vi "TestClone.vi"() -> ()   [LabVIEW 2014, in "EventModule.lvlib"]
uses:
  EventModule.lvlib
  EventPlugins/EventPluginBaseClass/TypeDefs/clEvtConfig.ctl
  PublicAPI/Arguments/Requests/dblEvtParams.ctl
  PublicAPI/Arguments/Requests/dblTimeArray.ctl
  EventPlugins/EventPluginBaseClass/TypeDefs/clEvtReportArray.ctl
  EventPlugins/EventPluginBaseClass/TypeDefs/clEvtReport.ctl
  EventPlugins/EventPluginBaseClass/TypeDefs/dblEvtSignalArray.ctl
  TestInfo.ctl
  <userlib>/NIST/ModuleAdminLib/ModuleAdmin/ModuleAdmin.lvclass
  PublicAPI/Arguments/Broadcasts/clDidInit.ctl
  <userlib>/NIST/ModuleAdminLib/ModuleAdmin/ModuleAdmin.lvclass/ModuleAdmin.ctl
  PublicAPI/Arguments/Requests/clStopArgument.ctl
  PublicAPI/Arguments/Broadcasts/clStatUpdate.ctl
  PublicAPI/Arguments/Broadcasts/clErrorRpt.ctl
  <userlib>/NIST/ModuleAdminLib/ModuleAdmin/Accessors/Read CloneRegRef.vi
  <vilib>/Analysis/1siggen.llb/Ramp Pattern by Delta.vi
  <userlib>/NIST/ModuleAdminLib/CloneRegistration/CloneRegistration.lvclass
  EventPlugins/EventPluginBaseClass/EventPluginBaseClass.lvclass
  <vilib>/Analysis/NI_AALBase.lvlib
panel:
  in  "Show Panel":bool=TRUE
  in  "End Time":dbl
  in  "Start Time":dbl
  in  "Plugin Type":u16(ring) items=["C37.118.1", "Frequency Ramp", "Modulation", "Ringdown", "Steady State", "Step", "60255Harm", "User1", "User2"]
  in  "btnGetEvtSignal":bool
  out "dblEventSignalArray":T1
  out "PathToPluginIniFileReport":path=path "P:/Framework/Events/EventPlugins/SSEvtPlugin/SteadyStateEventPlugin.ini"
  in  "btnReadPathToPlugin":bool
  in  "btnGetEvtReportArray":bool
  out "clEvtReportArray":T2 {"Synx" format="%#_4g"}
  in  "btnReadEvtParams":bool
  in  "btnWriteEvtParams":bool
  in  "btnReadTimeArray":bool
  in  "btnWriteTimeArray":bool
  out "dblTimeArrayReport":T4
  out "dblEvtParamsReport":T5
  out "dblTimeArray":T4=[0.0, 0.05, 0.1, 0.15000000000000002, 0.2]
  in  "dblEvtParams":T5=[[0.0, 0.34657, 0.69677, 1.297, 1.4569, 6.0606, 7.2288, 8.9506, 11.705, 18.574], [1000.0, 24.879, 55.751, 46.204, 36.867, 1.995, 0.82578, 1.5487, 1.8652, 1.6268], [0.0, 1.876, 0.28983, 1.5993, 2.6728, 3.9286, 1.2558, 3.3379, 3.6506, 7.1708], [0.0, -67.696, -60.912, 99.138, -123.76, 176.38, -149.46, -106.27, -18.535, -59.29], [0.0, 0.0, 0.58767, 0.6985, 1.3263, 2.7275, 7.1783, 8.122, 14.704, 15.622], [200.0, 31.231, 41.605, 48.38, 1.6511, 0.84175, 2.671, 0.64619, 0.78365, 0.6061], [0.0, 6.2405, 2.3071, 0.28998, 1.025, 3.6069, 15.284, 3.3041, 2.4034, 2.5242], [0.0, 180.0, 37.683, 113.63, 41.526, 4.7072, 5.0124, -177.41, -50.759, 41.697], [568.0, 0.0, 0.0, 0.0, 0.0, 0.0, 0.0, 0.0, 0.0, 0.0], [0.0, 0.0, 0.0, 0.0, 0.0, 0.0, 0.0, 0.0, 0.0, 0.0], [0.0, 0.0, 0.0, 0.0, 0.0, 0.0, 0.0, 0.0, 0.0, 0.0], [0.0, 0.0, 0.0, 0.0, 0.0, 0.0, 0.0, 0.0, 0.0, 0.0], [0.0, 0.0, 0.0, 0.0, 0.0, 0.0, 0.0, 0.0, 0.0, 0.0]]
  out "clEvtConfigReport":T6={"T0(UTC)"=0.0, "F0"=0.0, "Fs"=60, "FSamp"=0, "bPosSeq"=FALSE}
  in  "btnReadEvtConfig":bool
  in  "clEvtConfig":T6={"T0(UTC)"=0.0, "F0"=60.0, "Fs"=60, "FSamp"=960, "bPosSeq"=FALSE}
  in  "btnWriteEvtConfig":bool
  in  "btnLoadPlugin":bool
  in  "btnRemove":bool
  out "Status Log":string
  out "Active Modules (Array)":string[](array[string])
  in  "btnAdd":bool
  in  "btnStop":bool
  in  "Select Module":i32(ring)=-1 caption="Select Module to send Request" items=["All"=-1]
  # "Hidden"
  # "Visible"
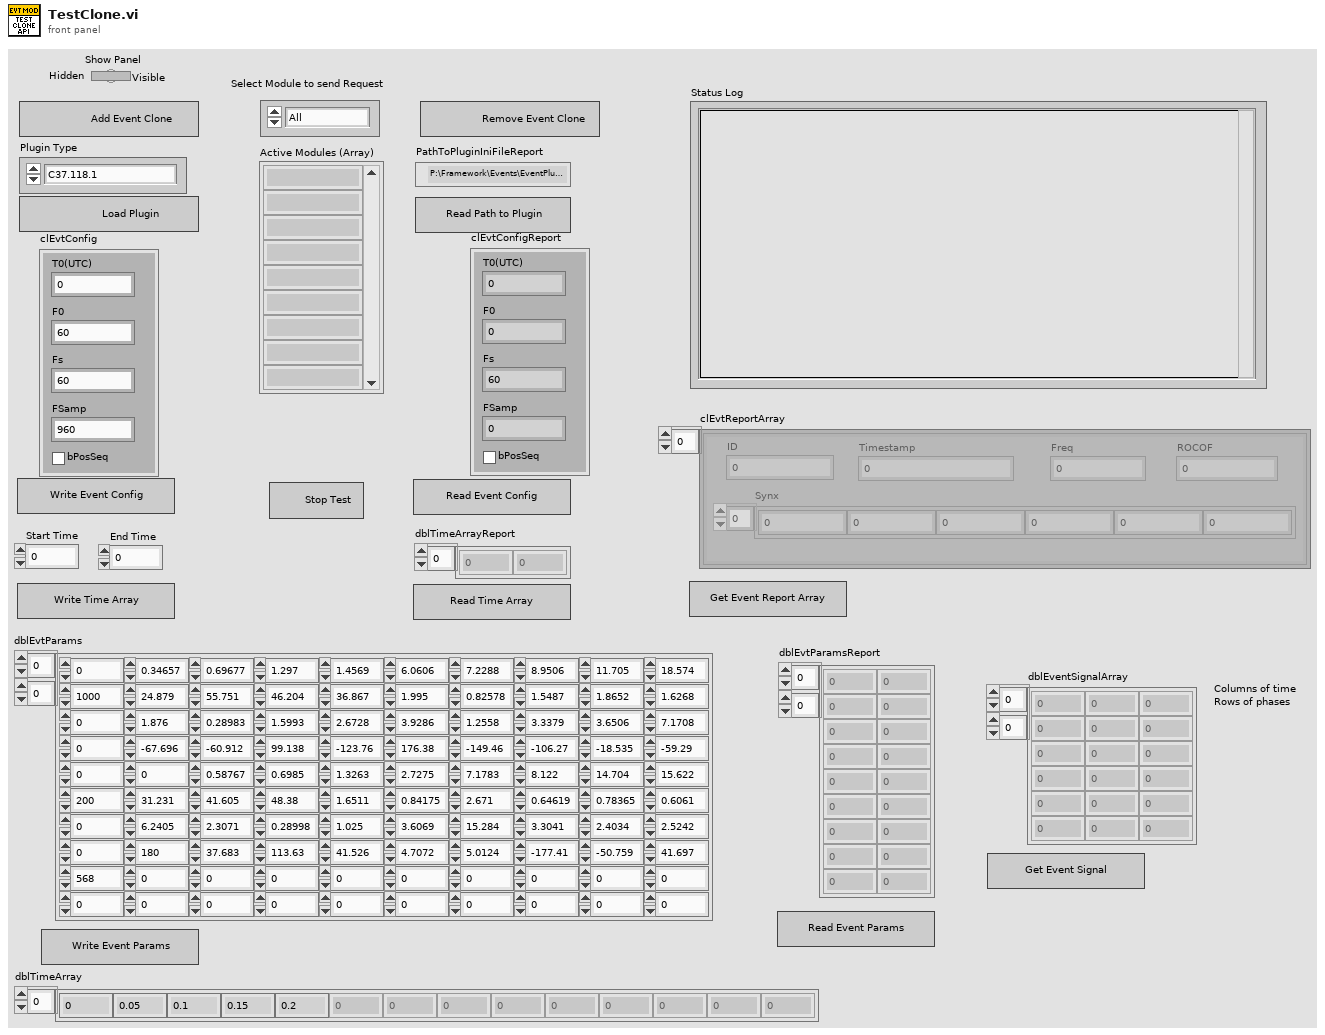
[diagram p1: front panel]
types:
  T1 = typedef "EventPlugins.lvlib/EventPluginBaseClass.lvclass/dblEvtSignalArray.ctl" = dbl[][]
  T2 = typedef "EventPlugins.lvlib/EventPluginBaseClass.lvclass/clEvtReportArray.ctl" = T3[]
  T3 = typedef "EventPlugins.lvlib/EventPluginBaseClass.lvclass/clEvtReport.ctl" = cluster{"Timestamp":dbl, "Synx":cdb[], "Freq":dbl, "ROCOF":dbl, "ID":i16}
  T4 = typedef "EventModule.lvlib/dblTimeArray.ctl" = dbl[]
  T5 = typedef "EventModule.lvlib/dblEvtParams.ctl" = dbl[][]
  T6 = typedef "EventPlugins.lvlib/EventPluginBaseClass.lvclass/clEvtConfig.ctl" = cluster{"T0(UTC)":dbl, "F0":dbl, "Fs":i32, "FSamp":u32, "bPosSeq":bool}
  T7 = typedef "EventModule.lvlib/TestInfo.ctl" = cluster{"PluginIniFilePaths":path[]}
  T8 = typedef "EventModule.lvlib/clBroadcastEvents.ctl" = cluster{"DidInit":refnum<user-event>, "StatusUpdate":refnum<user-event>, "ErrorReport":refnum<user-event>, "DidStop":refnum<user-event>, "ReadEvtConfig":refnum<user-event>, "ReadTimeArray":refnum<user-event>, "ReadEvtParams":refnum<user-event>, "GetEvtReportArray":refnum<user-event>, "ReadPathToPlugin":refnum<user-event>, "GetEvtSignal":refnum<user-event>, "ReadBusNumber":refnum<user-event>}
  T9 = typedef "EventModule.lvlib/clDidInit.ctl" = cluster{"Init?":bool, "ModuleAdmin":refnum<class "ModuleAdmin.lvclass">}
  T10 = typedef "EventModule.lvlib/clStopArgument.ctl" = cluster{"Exit via Stop Module Req?":bool, "Wait for Module to stop?":bool, "ModuleAdmin":refnum<class "ModuleAdmin.lvclass">}
  T11 = typedef "EventModule.lvlib/clStatUpdate.ctl" = cluster{"Status":string}
  T12 = typedef "EventModule.lvlib/clErrorRpt.ctl" = cluster{"error":errorcluster, "AdditionalInfo":string}
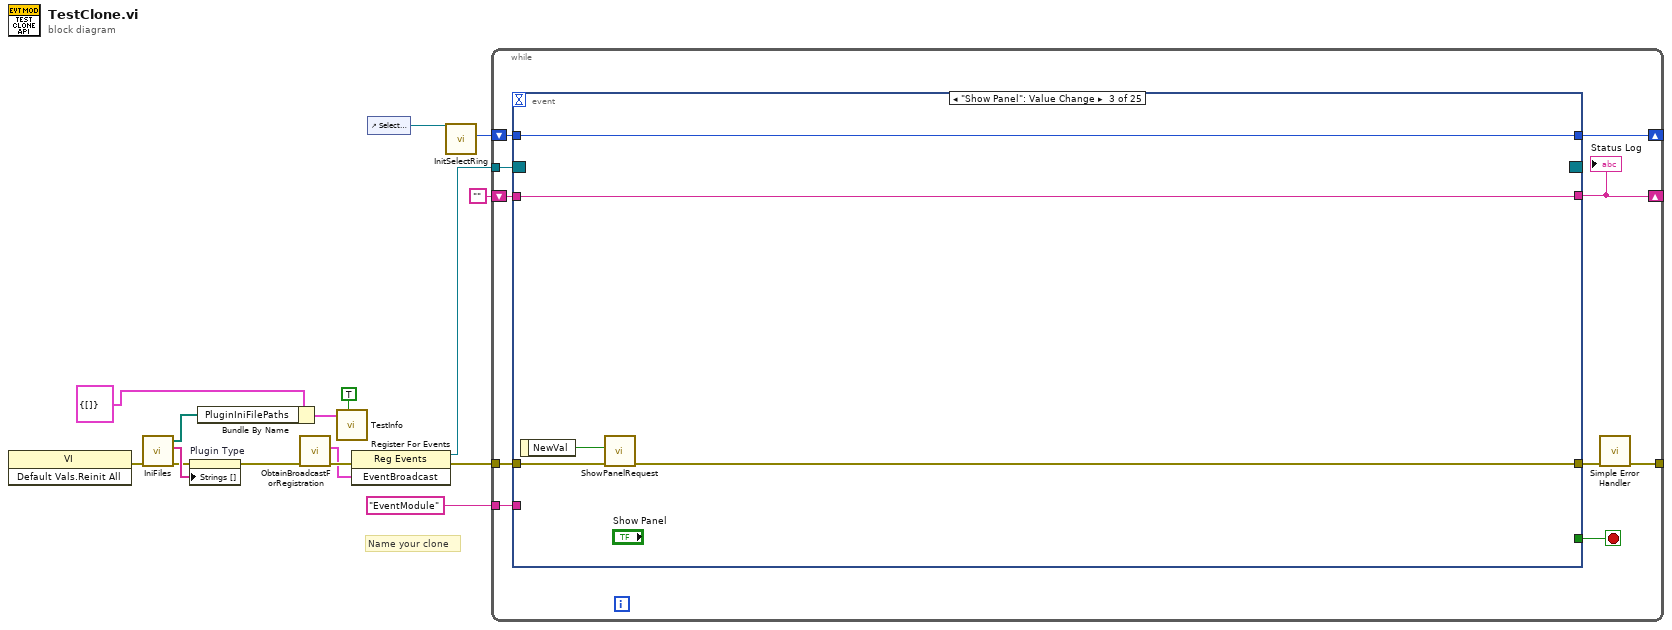
[diagram p0: block diagram]
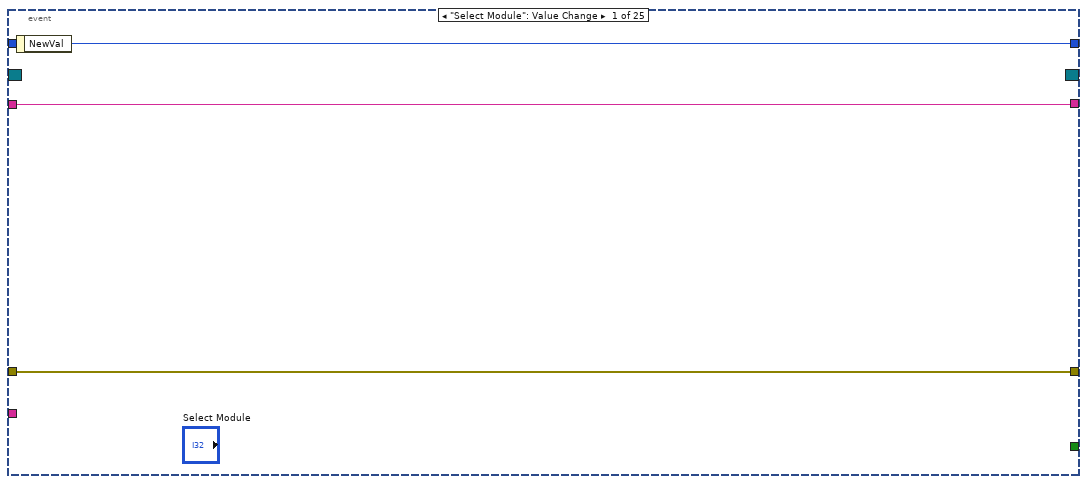
[diagram p2: hidden frame]
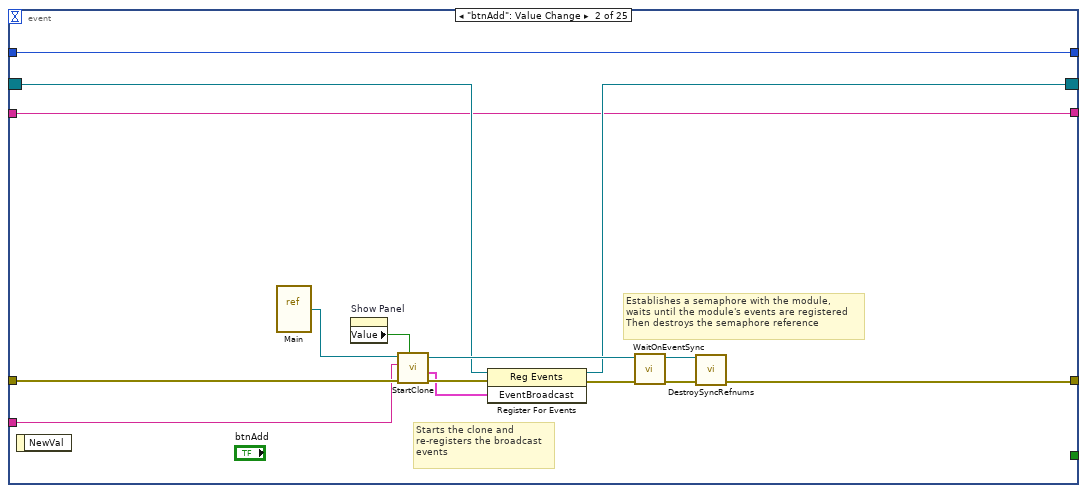
[diagram p3: hidden frame]
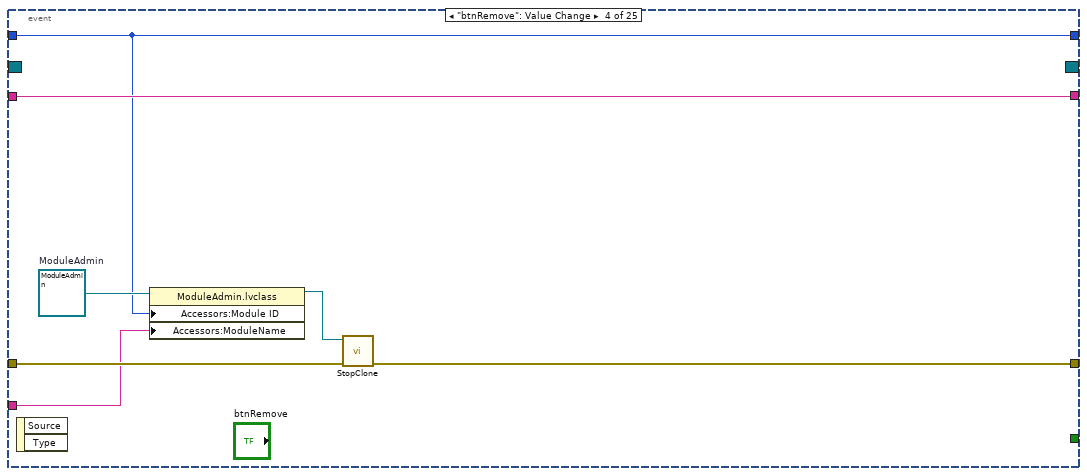
[diagram p4: hidden frame]
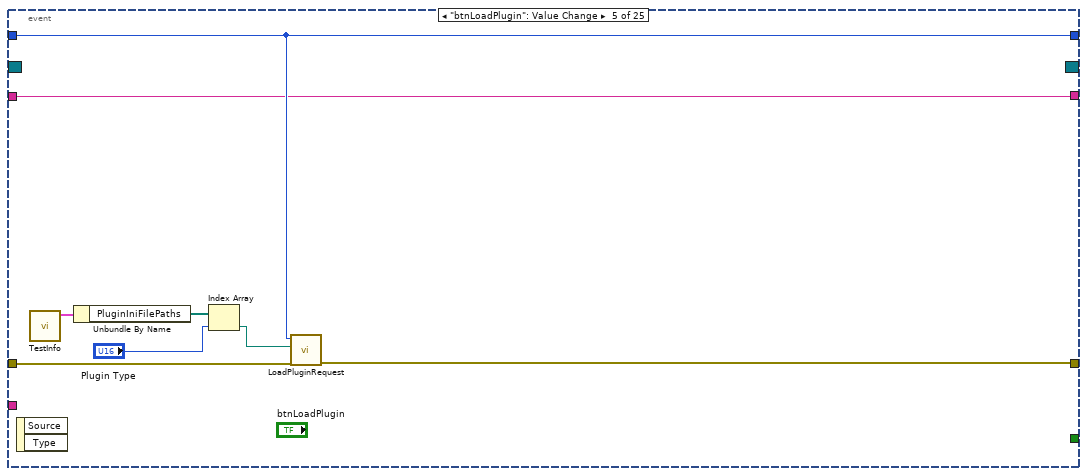
[diagram p5: hidden frame]
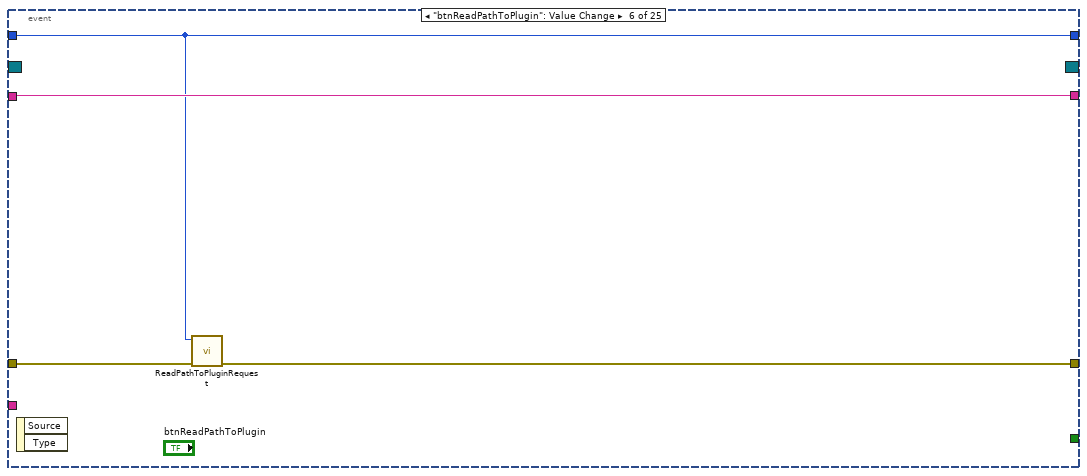
[diagram p6: hidden frame]
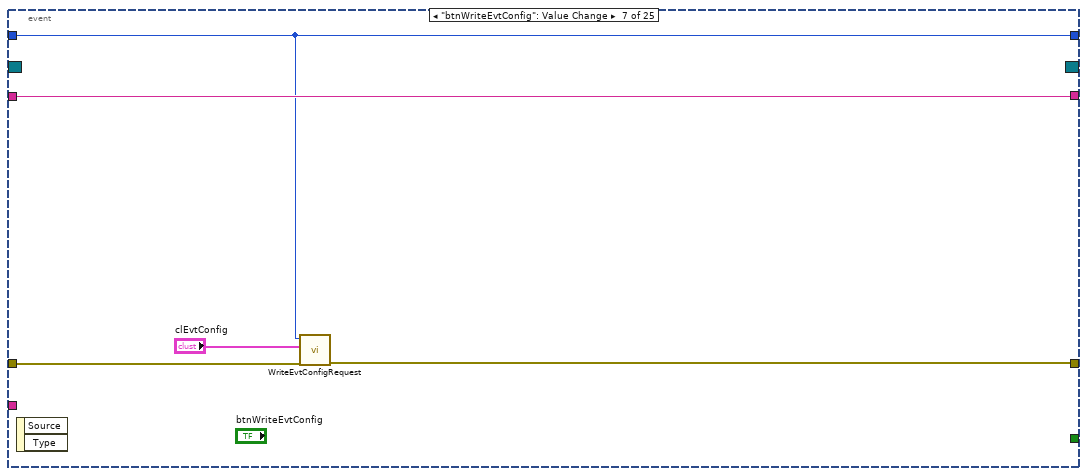
[diagram p7: hidden frame]
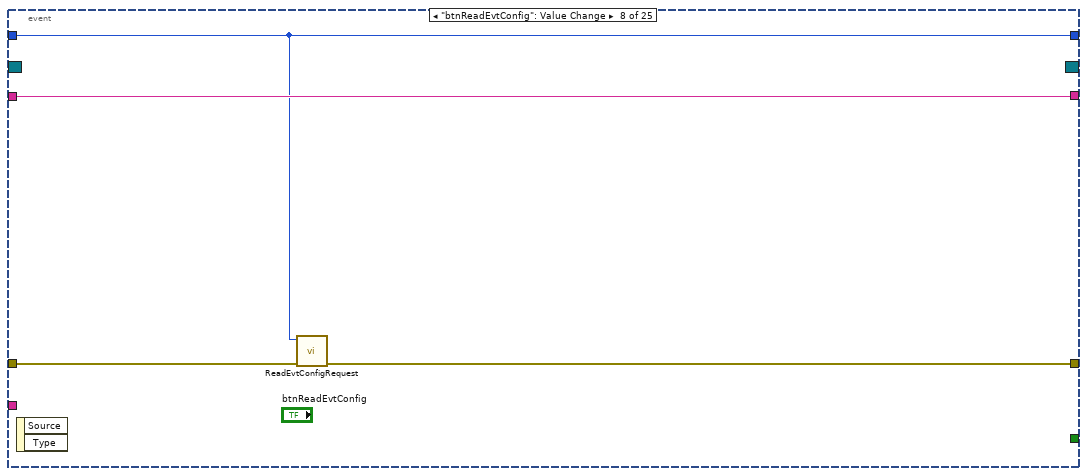
[diagram p8: hidden frame]
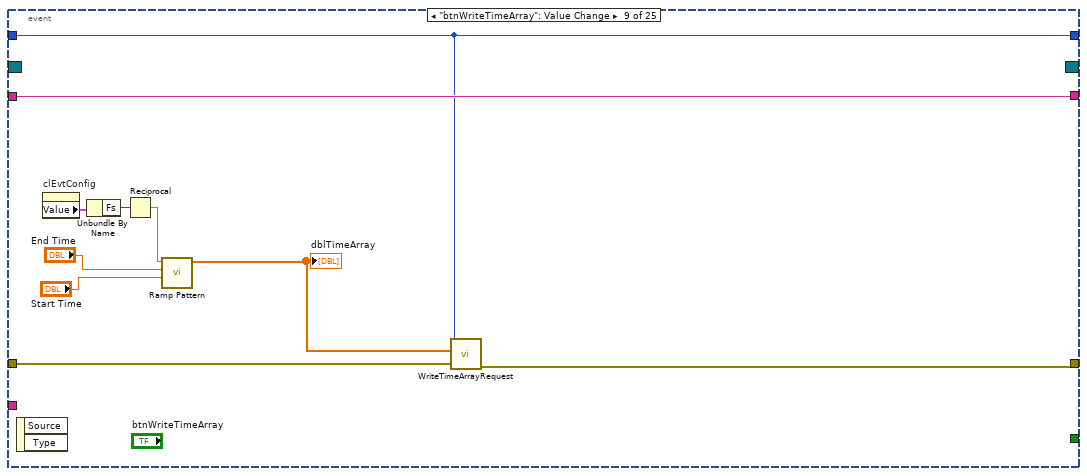
[diagram p9: hidden frame]
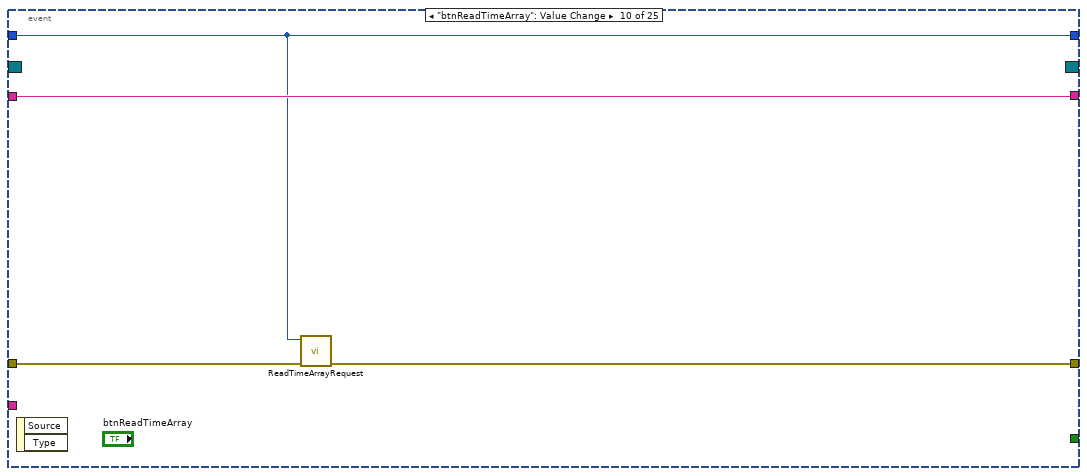
[diagram p10: hidden frame]
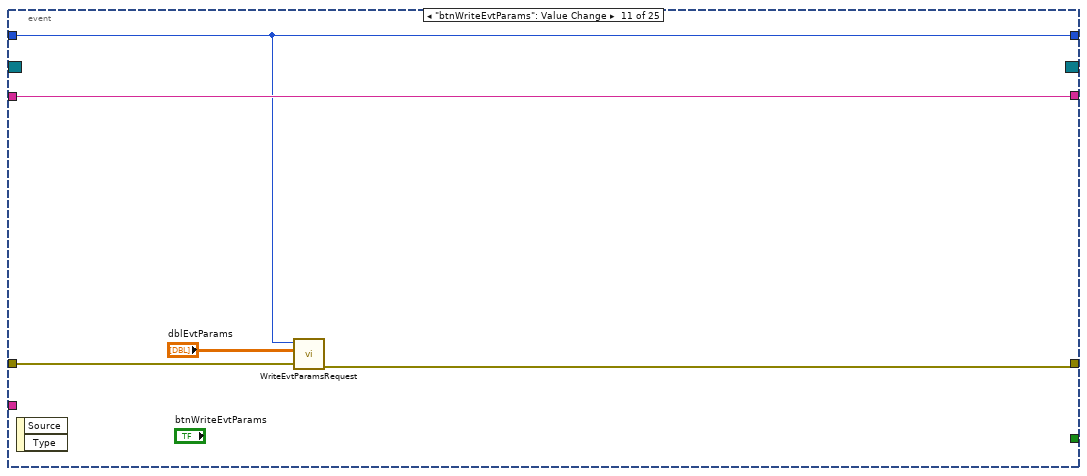
[diagram p11: hidden frame]
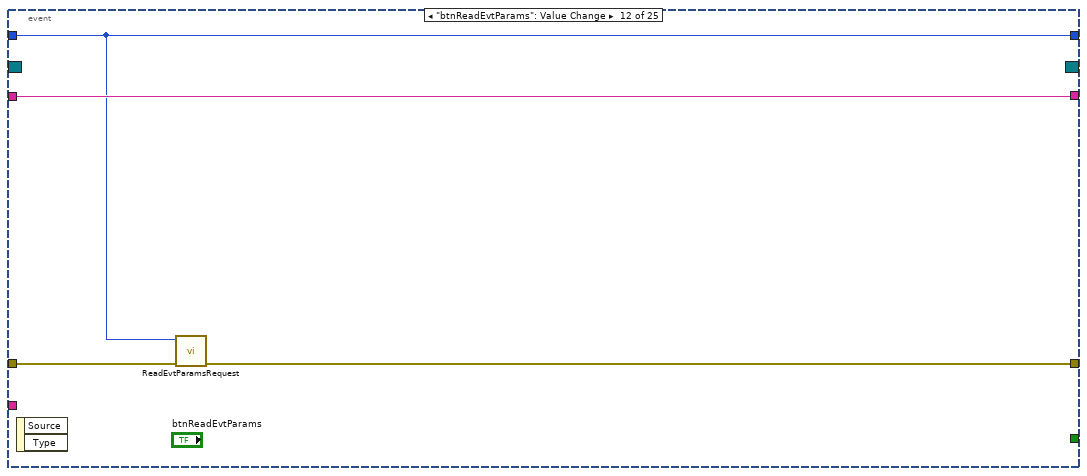
[diagram p12: hidden frame]
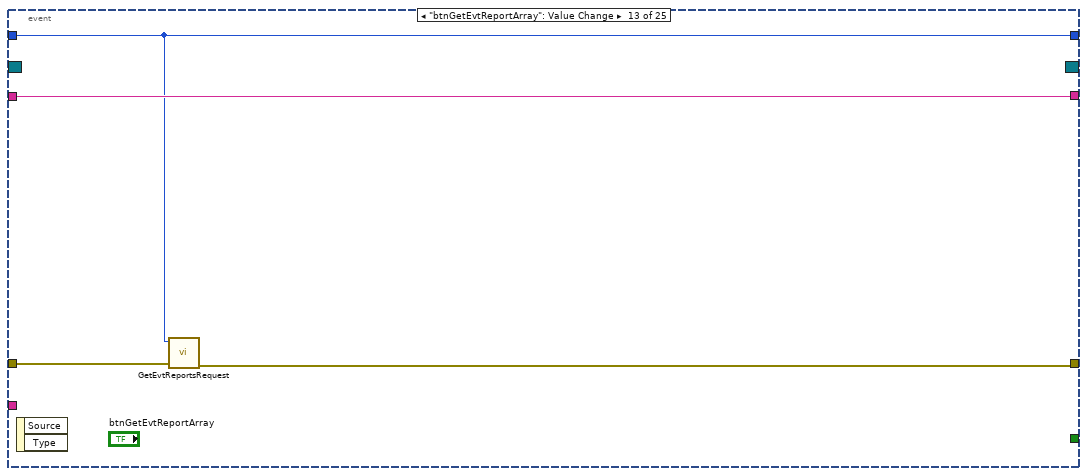
[diagram p13: hidden frame]
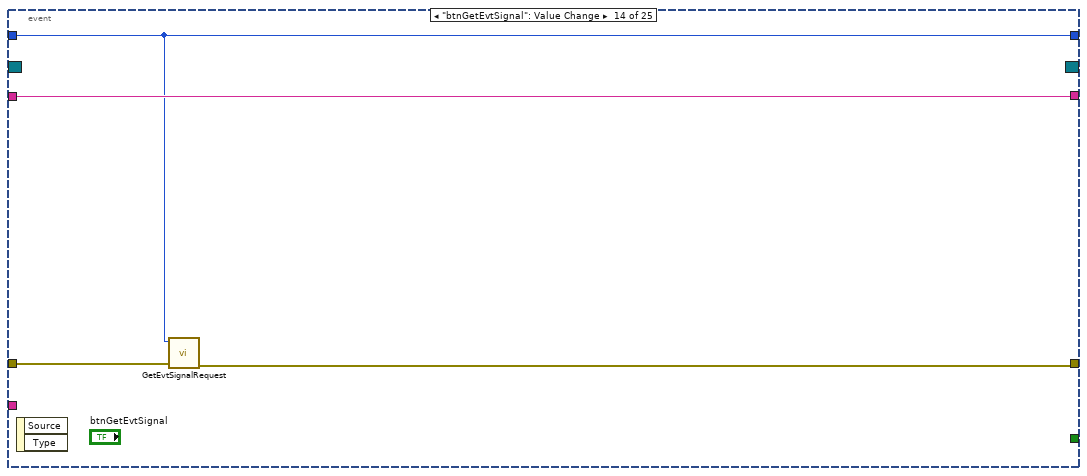
[diagram p14: hidden frame]
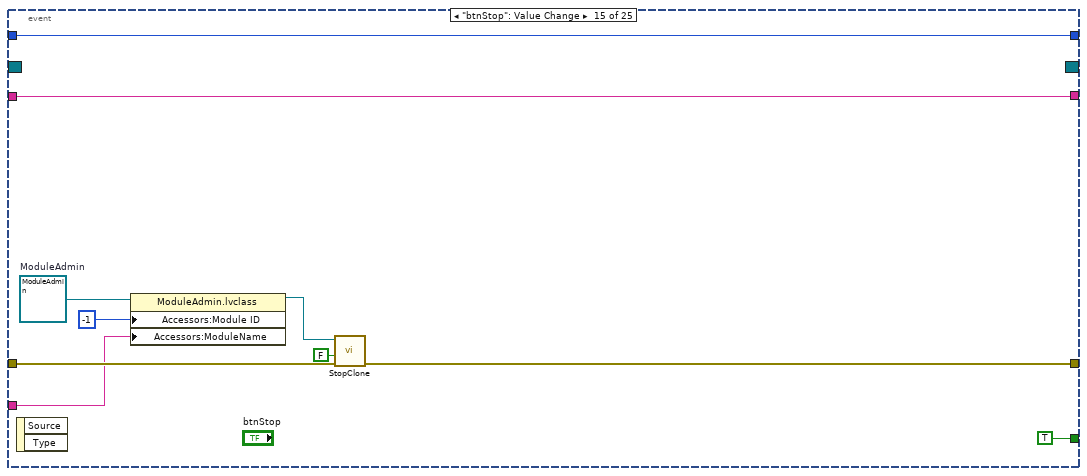
[diagram p15: hidden frame]
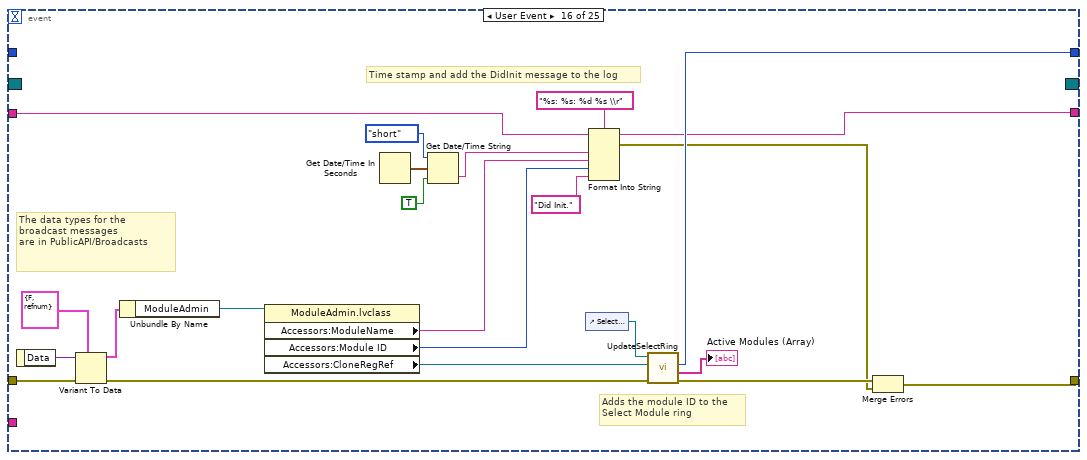
[diagram p16: hidden frame]
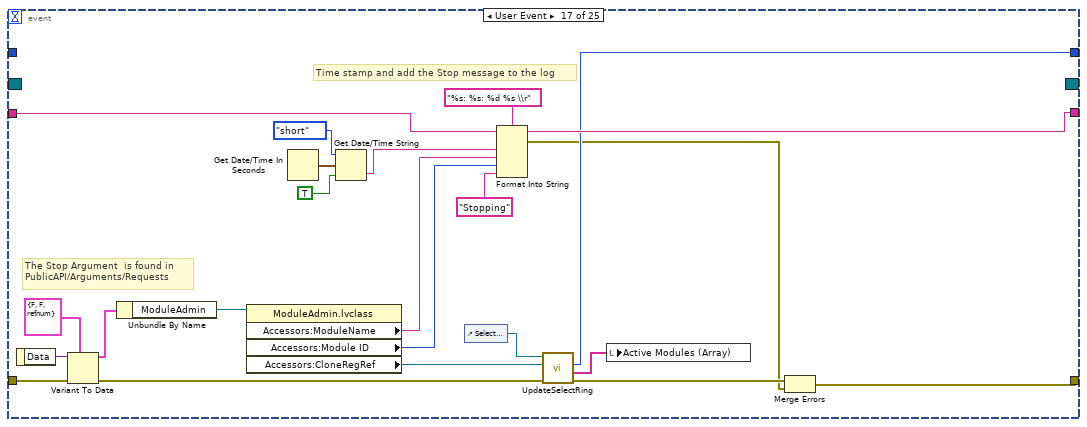
[diagram p17: hidden frame]
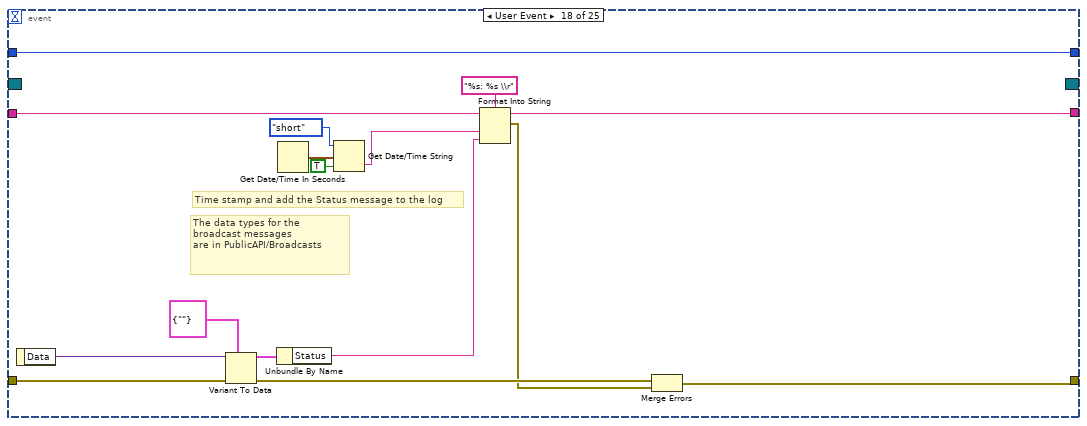
[diagram p18: hidden frame]
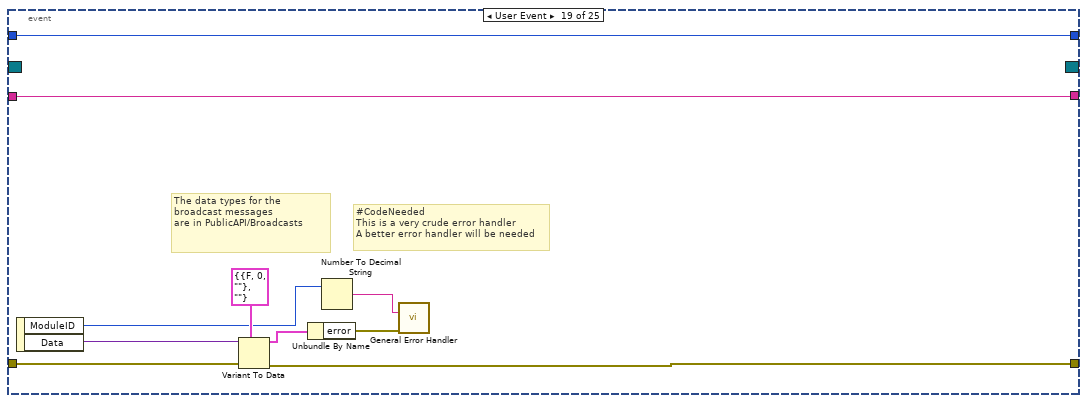
[diagram p19: hidden frame]
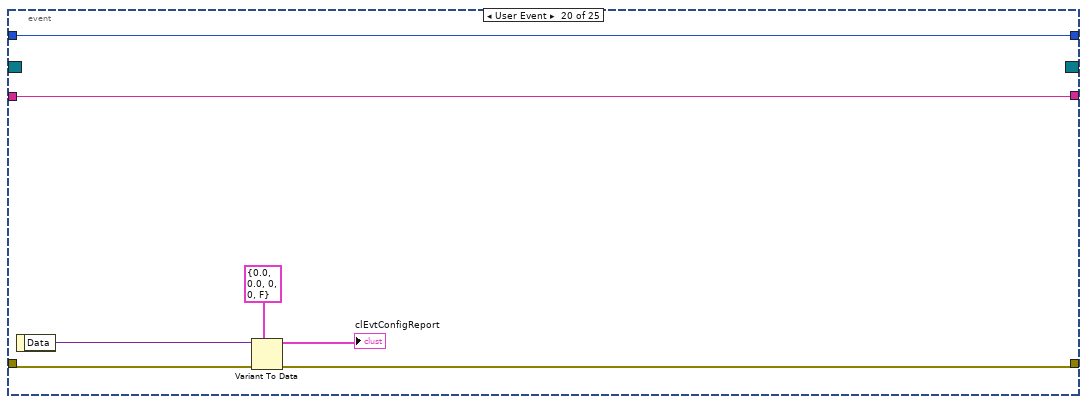
[diagram p20: hidden frame]
diagram:
  # "Name your clone"
  n1 = invoke class="VI" method="Default Vals.Reinit All"() -> (error out=w8:errorcluster)  [unwired: 3 in, 2 out]
  n2 = call "IniFiles.vi"("error in"=w8) -> ("error out"=w6:errorcluster, "Types"=w7:string[], "IniFilePaths"=w3:path[])  [unwired: 8 in]
  n3 = property on="Plugin Type" class="Ring (strict)"(error in=w6, "Strings []"=w7) -> (error out=w5:errorcluster)  [unwired: 1 in, 1 out]
  n4 = Bundle By Name(cluster=T7 {"PluginIniFilePaths"=[]} ("TestInfo"), "PluginIniFilePaths"=w3) -> (w2:T7)
  n5 = call "ObtainBroadcastForRegistration.vi"("error in (no error)"=w5) -> ("error out"=w14:errorcluster, "EventBroadcast"=w13:T8)  [unwired: 9 in]
  n6 = call "TestInfo.vi"("Set (f)"=TRUE, "TestInfo"=w2) -> ()  [unwired: 9 in, 1 out]
  n7 = register-events(error in=w14, w13) -> (reference out=w11:refnum<event-registration>, error out=w12:errorcluster)  [unwired: 1 in]
  n8 = control-ref of="Select Module"() -> (w16:refnum<vi>)
  n9 = call "InitSelectRing.vi"("Ring Refnum"=w16) -> ("Module Ring Value"=w15:i32)  [unwired: 9 in, 1 out]
  n10 = while {
    shift-right: [w25] -> _
    shift-left: w15 -> [w26]
    tunnel: w12 -> [w23]
    tunnel: w11 -> [w20]
    tunnel: [w21] -> _
    shift-right: [w19] -> _
    shift-left: "" -> [w18]
    tunnel: "EventModule" ("ModuleName") -> [w17]
    stop <- w24 stop-if-true
    n11 = event shown="[2] \"Show Panel\": Value Change" {
      selector: w20 -> [_ w35 _ _ _ _ _ _ _ _ _ _ _ _ _ _ _ _ _ _ _ _ _ _ _]
      dyn-events: [_ w34 _ _ _ _ _ _ _ _ _ _ _ _ _ _ _ _ _ _ _ _ _ _ _] -> _
      timeout: _ -> [_ _ _ _ _ _ _ _ _ _ _ _ _ _ _ _ _ _ _ _ _ _ _ _ _]
      tunnel: w26 -> [_ w44 w45 w51 w63 w65 w70 w74 w84 w90 w93 w98 w101 w105 w118 _ _ w180 w182 w191 w199 w206 w213 w220 w228]
      tunnel: [w29 w44 w45 w51 w63 w65 w70 w74 w84 w90 w93 w98 w101 w105 w118 w136 w151 w180 w182 w191 w199 w206 w213 w220 w228] -> w25
      tunnel: [_ _ _ _ _ _ _ _ _ _ _ _ _ _ TRUE _ _ _ _ _ _ _ _ _ _] -> w24
      tunnel: w23 -> [w27 w43 w49 w55 w64 w67 w72 w76 w87 w89 w96 w99 w104 w108 w116 w141 w160 w177 w189 w194 w204 w208 w217 w225 w232]
      tunnel: [w27 w36 w47 w54 w62 w66 w69 w75 w86 w88 w94 w97 w103 w107 w114 w124 w148 w168 w188 w193 w203 w209 w215 w224 w231] -> w22
      tunnel: [w28 w32 w46 w56 w61 w68 w73 w77 w85 w91 w95 w100 w102 w106 w113 w128 w157 w171 w181 w192 w198 w207 w214 w221 w229] -> w19
      tunnel: w18 -> [w28 w32 w46 w56 w61 w68 w73 w77 w85 w91 w95 w100 w102 w106 w113 w127 w158 w179 w181 w192 w198 w207 w214 w221 w229]
      tunnel: w17 -> [_ w31 _ w52 _ _ _ _ _ _ _ _ _ _ w110 _ _ _ _ _ _ _ _ _ _]
      event "Select Module": Value Change {
        n12 = event-data() -> ("NewVal"=w29:i32)  [unwired: 1 in]
      }
      event "btnAdd": Value Change {
        # "Establishes a semaphore with the module,\nwaits until the module's events are registered\nThen destroys the semaphore reference"
        # "Starts the clone and\nre-registers the broadcast \nevents"
        n13 = event-data() -> ()  [unwired: 1 in, 1 out]
        n14 = vi-ref "Main.vi"() -> (w33:refnum<vi>)
        n15 = property on="Show Panel" class="Bool (strict)"() -> ("Value"=w30:bool)  [unwired: 2 in, 2 out]
        n16 = call "StartClone.vi"("ShowPanel? (f)"=w30, "error in (no error)"=w43, "ModuleName"=w31, "VI Refnum"=w33) -> ("error out"=w42:errorcluster, "clBroadcastEvents"=w37:T8, "ModuleAdmin"=w39:refnum<class "ModuleAdmin.lvclass">)  [unwired: 5 in]
        n17 = register-events(reference=w35, error in=w42, w37) -> (reference out=w34:refnum<event-registration>, error out=w41:errorcluster)
        n18 = call <userlib>:"WaitOnEventSync.vi"("error in (no error)"=w41, "ModuleAdmin"=w39) -> ("error out"=w40:errorcluster, "ModuleAdmin"=w38:refnum<class "ModuleAdmin.lvclass">)  [unwired: 8 in]
        n19 = call <userlib>:"DestroySyncRefnums.vi"("error in (no error)"=w40, "ModuleAdmin"=w38) -> ("error out"=w36:errorcluster)  [unwired: 9 in]
      }
      event "Show Panel": Value Change {
        n20 = event-data() -> ("NewVal"=w48:bool)  [unwired: 1 in]
        n21 = call "ShowPanelRequest.vi"("error in (no error)"=w49, "ShowPanel?"=w48) -> ("error out"=w47:errorcluster)  [unwired: 9 in]
      }
      event "btnRemove": Value Change {
        w53 = refnum<class "ModuleAdmin.lvclass"> refnum  # ModuleAdmin
        n22 = event-data() -> ()  [unwired: 1 in, 2 out]
        n23 = property class="ModuleAdmin.lvclass"(reference=w53, "Accessors:Module ID"=w51, "Accessors:ModuleName"=w52) -> (reference out=w50:refnum<class "ModuleAdmin.lvclass">)  [unwired: 1 in, 1 out]
        n24 = call "StopClone.vi"("error in (no error)"=w55, "ModuleAdmin"=w50) -> ("error out"=w54:errorcluster)  [unwired: 9 in]
      }
      event "btnLoadPlugin": Value Change {
        n25 = event-data() -> ()  [unwired: 1 in, 2 out]
        n26 = call "TestInfo.vi"() -> ("TestInfo"=w60:T7)  [unwired: 11 in]
        n27 = Unbundle By Name(w60) -> ("PluginIniFilePaths"=w59:path[])
        n28 = Index Array(array=w59, index="Plugin Type") -> (element=w57:path)
        n29 = call "LoadPluginRequest.vi"("error in (no error)"=w64, "PathToPlugin"=w57, "ModuleID"=w63) -> ("error out"=w62:errorcluster)  [unwired: 8 in]
      }
      event "btnReadPathToPlugin": Value Change {
        n30 = event-data() -> ()  [unwired: 1 in, 2 out]
        n31 = call "ReadPathToPluginRequest.vi"("error in (no error)"=w67, "ModuleID"=w65) -> ("error out"=w66:errorcluster)  [unwired: 9 in]
      }
      event "btnWriteEvtConfig": Value Change {
        n32 = event-data() -> ()  [unwired: 1 in, 2 out]
        n33 = call "WriteEvtConfigRequest.vi"("error in (no error)"=w72, "clEvtConfig"="clEvtConfig", "ModuleID"=w70) -> ("error out"=w69:errorcluster)  [unwired: 8 in]
      }
      event "btnReadEvtConfig": Value Change {
        n34 = event-data() -> ()  [unwired: 1 in, 2 out]
        n35 = call "ReadEvtConfigRequest.vi"("error in (no error)"=w76, "ModuleID"=w74) -> ("error out"=w75:errorcluster)  [unwired: 9 in]
      }
      event "btnWriteTimeArray": Value Change {
        n36 = event-data() -> ()  [unwired: 1 in, 2 out]
        n37 = property on="clEvtConfig" class="Clust (strict)"() -> ("Value"=w81:T6)  [unwired: 2 in, 2 out]
        n38 = Unbundle By Name(w81) -> ("Fs"=w80:i32)
        n39 = Reciprocal(x=w80) -> (1/x=w79:dbl)
        n40 = call-poly <vilib>:"Ramp Pattern.vi"("start"="Start Time", "end"="End Time", "delta"=w79) -> ("Ramp Pattern"=w78:dbl[])  [unwired: 6 in, 2 out]
        "dblTimeArray" <- w78
        n41 = call "WriteTimeArrayRequest.vi"("error in (no error)"=w87, "TimeArray"=w78, "ModuleID"=w84) -> ("error out"=w86:errorcluster)  [unwired: 8 in]
      }
      event "btnReadTimeArray": Value Change {
        n42 = event-data() -> ()  [unwired: 1 in, 2 out]
        n43 = call "ReadTimeArrayRequest.vi"("error in (no error)"=w89, "ModuleID"=w90) -> ("error out"=w88:errorcluster)  [unwired: 9 in]
      }
      event "btnWriteEvtParams": Value Change {
        n44 = event-data() -> ()  [unwired: 1 in, 2 out]
        n45 = call "WriteEvtParamsRequest.vi"("error in (no error)"=w96, "EvtParams"="dblEvtParams", "ModuleID"=w93) -> ("error out"=w94:errorcluster)  [unwired: 8 in]
      }
      event "btnReadEvtParams": Value Change {
        n46 = event-data() -> ()  [unwired: 1 in, 2 out]
        n47 = call "ReadEvtParamsRequest.vi"("error in (no error)"=w99, "ModuleID"=w98) -> ("error out"=w97:errorcluster)  [unwired: 9 in]
      }
      event "btnGetEvtReportArray": Value Change {
        n48 = event-data() -> ()  [unwired: 1 in, 2 out]
        n49 = call "GetEvtReportsRequest.vi"("error in (no error)"=w104, "ModuleID"=w101) -> ("error out"=w103:errorcluster)  [unwired: 9 in]
      }
      event "btnGetEvtSignal": Value Change {
        n50 = event-data() -> ()  [unwired: 1 in, 2 out]
        n51 = call "GetEvtSignalRequest.vi"("error in (no error)"=w108, "ModuleID"=w105) -> ("error out"=w107:errorcluster)  [unwired: 9 in]
      }
      event "btnStop": Value Change {
        w112 = refnum<class "ModuleAdmin.lvclass"> refnum  # ModuleAdmin
        n52 = event-data() -> ()  [unwired: 1 in, 2 out]
        n53 = property class="ModuleAdmin.lvclass"(reference=w112, "Accessors:Module ID"=-1 ("Module ID"), "Accessors:ModuleName"=w110) -> (reference out=w109:refnum<class "ModuleAdmin.lvclass">)  [unwired: 1 in, 1 out]
        n54 = call "StopClone.vi"("error in (no error)"=w116, "Wait for Module to stop?"=FALSE, "ModuleAdmin"=w109) -> ("error out"=w114:errorcluster)  [unwired: 8 in]
      }
      event User Event {
        # "Adds the module ID to the \nSelect Module ring"
        # "Time stamp and add the DidInit message to the log"
        # "The data types for the broadcast messages\nare in PublicAPI/Broadcasts"
        n55 = event-data() -> ("Data"=w140:variant)  [unwired: 1 in]
        n56 = Variant To Data(error in=w141, type=T9 {"Init?"=FALSE, "ModuleAdmin"=refnum} ("clDidInit"), Variant=w140) -> (data=w133:T9, error out=w138:errorcluster)
        n57 = Unbundle By Name(w133) -> ("ModuleAdmin"=w132:refnum<class "ModuleAdmin.lvclass">)
        n58 = property class="ModuleAdmin.lvclass"(reference=w132) -> ("Accessors:ModuleName"=w121:string, "Accessors:Module ID"=w120:i32, "Accessors:CloneRegRef"=w119:refnum<data-value>)  [unwired: 1 in, 2 out]
        n59 = Get Date/Time In Seconds() -> (seconds since 1Jan1904=w130:timestamp)
        n60 = Get Date/Time String(date format (0)=enum16{"short", "long", "abbreviated"}."short", seconds (now)=w130, want seconds? (F)=TRUE) -> (time string=w134:string)  [unwired: 1 out]
        n61 = control-ref of="Select Module"() -> (w137:refnum<vi>)
        n62 = Format Into String(format string="%s: %s: %d %s \\r", initial string=w127, w134, w121, w120, "Did Init.") -> (resulting string=w128:string, error out=w125:errorcluster)  [unwired: 1 in]
        n63 = call "UpdateSelectRing.vi"("error in (no error)"=w138, "CloneRegRef"=w119, "Ring Refnum"=w137) -> ("error out"=w126:errorcluster, "ActiveModules"=→"Active Modules (Array)":string[], "Module Ring Value"=w136:i32)  [unwired: 6 in]
        n64 = Merge Errors(w126, w125) -> (w124:errorcluster)
      }
      event User Event {
        # "Time stamp and add the Stop message to the log"
        # "The Stop Argument  is found in\nPublicAPI/Arguments/Requests"
        n65 = event-data() -> ("Data"=w159:variant)  [unwired: 1 in]
        n66 = Variant To Data(error in=w160, type=T10 {"Exit via Stop Module Req?"=FALSE, "Wait for Module to stop?"=FALSE, "ModuleAdmin"=refnum} ("Stop Argument"), Variant=w159) -> (data=w155:T10, error out=w154:errorcluster)
        n67 = Unbundle By Name(w155) -> ("ModuleAdmin"=w146:refnum<class "ModuleAdmin.lvclass">)
        n68 = property class="ModuleAdmin.lvclass"(reference=w146) -> ("Accessors:ModuleName"=w143:string, "Accessors:Module ID"=w142:i32, "Accessors:CloneRegRef"=w145:refnum<data-value>)  [unwired: 1 in, 2 out]
        n69 = Get Date/Time In Seconds() -> (seconds since 1Jan1904=w162:timestamp)
        n70 = Get Date/Time String(date format (0)=enum16{"short", "long", "abbreviated"}."short", seconds (now)=w162, want seconds? (F)=TRUE) -> (time string=w164:string)  [unwired: 1 out]
        n71 = control-ref of="Select Module"() -> (w153:refnum<vi>)
        n72 = Format Into String(format string="%s: %s: %d %s \\r", initial string=w158, w164, w143, w142, "Stopping") -> (resulting string=w157:string, error out=w149:errorcluster)  [unwired: 1 in]
        n73 = call "UpdateSelectRing.vi"("error in (no error)"=w154, "CloneRegRef"=w145, "Ring Refnum"=w153) -> ("error out"=w150:errorcluster, "ActiveModules"=w152:string[], "Module Ring Value"=w151:i32)  [unwired: 6 in]
        n74 = local write "Active Modules (Array)"(w152) -> ()
        n75 = Merge Errors(w150, w149) -> (w148:errorcluster)
      }
      event User Event {
        # "Time stamp and add the Status message to the log"
        # "The data types for the broadcast messages\nare in PublicAPI/Broadcasts"
        n76 = event-data() -> ("Data"=w176:variant)  [unwired: 1 in]
        n77 = Variant To Data(error in=w177, type=T11 {"Status"=""} ("clStatUpdate"), Variant=w176) -> (data=w174:T11, error out=w170:errorcluster)
        n78 = Unbundle By Name(w174) -> ("Status"=w172:string)
        n79 = Get Date/Time In Seconds() -> (seconds since 1Jan1904=w173:timestamp)
        n80 = Get Date/Time String(date format (0)=enum16{"short", "long", "abbreviated"}."short", seconds (now)=w173, want seconds? (F)=TRUE) -> (time string=w165:string)  [unwired: 1 out]
        n81 = Format Into String(format string="%s: %s \\r", initial string=w179, w165, w172) -> (resulting string=w171:string, error out=w169:errorcluster)  [unwired: 1 in]
        n82 = Merge Errors(w170, w169) -> (w168:errorcluster)
      }
      event User Event {
        # "#CodeNeeded\nThis is a very crude error handler\nA better error handler will be needed"
        # "The data types for the broadcast messages\nare in PublicAPI/Broadcasts"
        n83 = event-data() -> ("ModuleID"=w185:i32, "Data"=w190:variant)  [unwired: 1 in]
        n84 = Variant To Data(error in=w189, type=T12 {"error"={"status"=FALSE, "code"=0, "source"=""}, "AdditionalInfo"=""} ("Cluster"), Variant=w190) -> (data=w186:T12, error out=w188:errorcluster)
        n85 = Unbundle By Name(w186) -> ("error"=w184:errorcluster)
        n86 = Number To Decimal String(number=w185) -> (decimal integer string=w183:string)  [unwired: 1 in]
        n87 = call <vilib>:"General Error Handler.vi"("[error source] (\" \")"=w183, "error in (no error)"=w184) -> ()  [unwired: 9 in, 5 out]
      }
      event User Event {
        n88 = event-data() -> ("Data"=w197:variant)  [unwired: 1 in]
        n89 = Variant To Data(error in=w194, type=T6 {"T0(UTC)"=0.0, "F0"=0.0, "Fs"=0, "FSamp"=0, "bPosSeq"=FALSE} ("clEvtConfig"), Variant=w197) -> (data=→"clEvtConfigReport":T6, error out=w193:errorcluster)
      }
      event User Event {
        w200 = T4 []  # TimeArray
        n90 = event-data() -> ("Data"=w201:variant)  [unwired: 1 in]
        n91 = Variant To Data(error in=w204, type=w200, Variant=w201) -> (data=→"dblTimeArrayReport":T4, error out=w203:errorcluster)
      }
      event User Event {
        w211 = T5 []  # SignalParams
        n92 = event-data() -> ("Data"=w205:variant)  [unwired: 1 in]
        n93 = Variant To Data(error in=w208, type=w211, Variant=w205) -> (data=→"dblEvtParamsReport":T5, error out=w209:errorcluster)
      }
      event User Event {
        n94 = event-data() -> ("Data"=w218:variant)  [unwired: 1 in]
        n95 = Variant To Data(error in=w217, type=path "", Variant=w218) -> (data=→"PathToPluginIniFileReport":path, error out=w215:errorcluster)
      }
      event User Event {
        w219 = T2 []  # ReportArray
        n96 = event-data() -> ("Data"=w223:variant)  [unwired: 1 in]
        n97 = Variant To Data(error in=w225, type=w219, Variant=w223) -> (data=→"clEvtReportArray":T2, error out=w224:errorcluster)
      }
      event User Event {
        n98 = event-data() -> ("Data"=w230:variant)  [unwired: 1 in]
        n99 = Variant To Data(error in=w232, type=T1 [] ("dblEventSignalArray"), Variant=w230) -> (data=→"dblEventSignalArray":T1, error out=w231:errorcluster)
      }
    }
    "Status Log" <- w19
    n100 = call <vilib>:"Simple Error Handler.vi"("error in (no error)"=w22) -> ("error out"=w21:errorcluster)  [unwired: 4 in, 4 out]
  }
